vi "Setup.vi"(5 "Description":string, 7 "Name":string, 8 "error in (no error)":errorcluster, 9 "Version":string, 11 "Arguments":T1[](array[typedef]) {"Number" items=["? One or none"=0, "* Any"=-1, "+ At least one"=-2]}) -> (0 "error out":errorcluster, 3 "LV Argument Parser out":refnum<class "LV Argument Parser.lvclass">)   [LabVIEW 2023, in "LV ArgParse.lvlib" / "LV Argument Parser.lvclass"]
uses:
  LV Argument Parser.lvclass
  Argument Definition.ctl
  Program Info.ctl
  LV Argument Parser.lvclass/LV Argument Parser.ctl
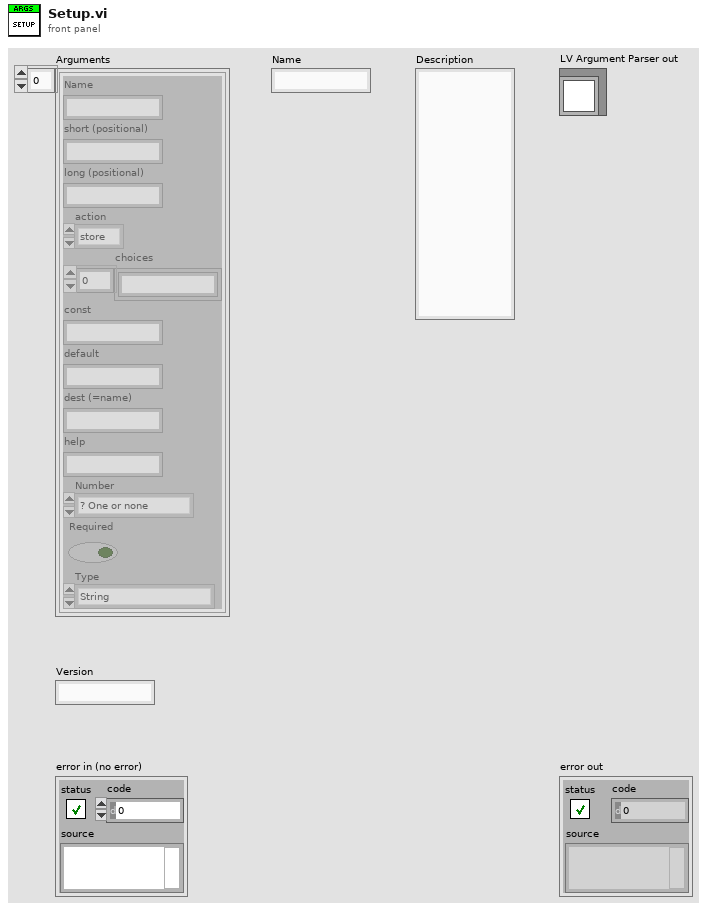
[diagram p1: front panel]
types:
  T1 = typedef "LV ArgParse.lvlib/LV Argument Parser.lvclass/Argument Definition.ctl" = cluster{"Name":string, "short (positional)":string, "long (positional)":string, "action":enum16{"store", "store-const", "store-false", "store-true", "append", "append-const", "count", "help", "version"}, "choices":string[], "const":string, "default":string, "dest (=name)":string, "help":string, "Number":i32, "Required":bool, "Type":enum16{"String", "Int", "Uint", "Float", "Bool", "Date", "Path"}}
  T2 = typedef "LV ArgParse.lvlib/LV Argument Parser.lvclass/Program Info.ctl" = cluster{"Name":string, "Description":string, "Version":string}
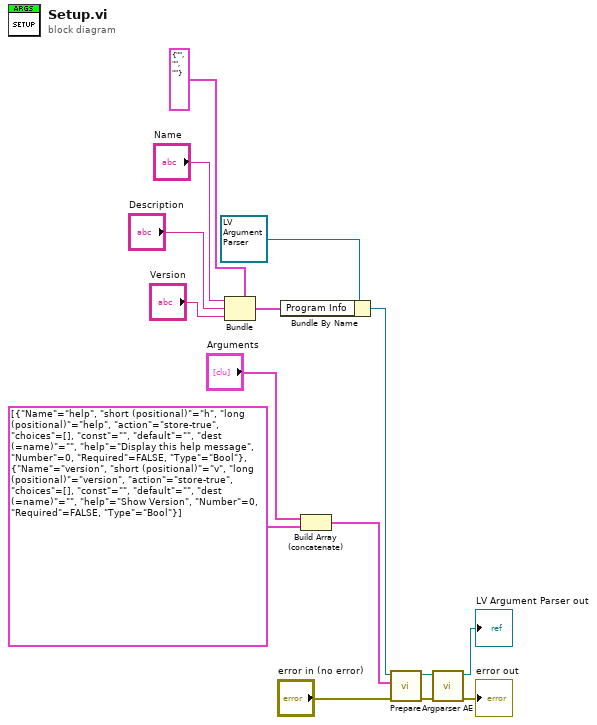
[diagram p0: block diagram]
diagram:
  n1 = Bundle(cluster=T2 {"Name"="", "Description"="", "Version"=""} ("Program Info"), "Name"="Name", "Description"="Description", "Version"="Version") -> (w7:T2)
  n2 = Bundle By Name(cluster=refnum<class "LV Argument Parser.lvclass"> refnum ("LV Argument Parser in"), "Program Info"=w7) -> (w8:refnum<class "LV Argument Parser.lvclass">)
  n3 = Build Array (concatenate)("Arguments", T1[] [{"Name"="help", "short (positional)"="h", "long (positional)"="help", "action"=enum."store-true", "choices"=[], "const"="", "default"="", "dest (=name)"="", "help"="Display this help message", "Number"=0, "Required"=FALSE, "Type"=enum."Bool"}, {"Name"="version", "short (positional)"="v", "long (positional)"="version", "action"=enum."store-true", "choices"=[], "const"="", "default"="", "dest (=name)"="", "help"="Show Version", "Number"=0, "Required"=FALSE, "Type"=enum."Bool"}] ("Array")) -> (w4:T1[])
  n4 = call "Prepare.vi"("error in (no error)"="error in (no error)", "Arguments"=w4, "LV Argument Parser in"=w8) -> ("error out"=w14:errorcluster, "LV Argument Parser out"=w10:refnum<class "LV Argument Parser.lvclass">)  [unwired: 7 in]
  n5 = call "Argparser AE.vi"("error in (no error)"=w14, "LV Argument Parser in"=w10) -> ("error out"=→"error out":errorcluster, "LV Argument Parser out"=→"LV Argument Parser out":refnum<class "LV Argument Parser.lvclass">)  [unwired: 8 in]
